vi "Actor Core.vi"(8 "error in":errorcluster, 11 "CS++BaseActor in":refnum<class "CS++BaseActor.lvclass">) -> (0 "error out":errorcluster, 3 "Actor out":refnum<class "Actor.lvclass">)   [LabVIEW 2016, in "CS++BaseActor.lvlib" / "CS++BaseActor.lvclass"]
doc: "(<B>Filename</B>: Actor Framework.lvlib:Actor.lvclass:Actor Core.vi)\n\nReceives messages to the actor, reacts to them, and initiates any error handling that may shut the actor down.\n\nDescendant classes may override this VI to append parallel tasks for the actor to complete while it handles messages. Overrides use the Call Parent Method node."
uses:
  CS++BaseActor.lvclass
  C:/Program Files (x86)/National Instruments/LabVIEW 2016/vi.lib/ActorFramework/Actor/Actor.lvclass
  <vilib>/ActorFramework/Actor/Actor.lvclass
  CS++BaseActor.lvclass/CS++BaseActor.ctl
  <vilib>/ActorFramework/Message Enqueuer/Message Priority.ctl
  <vilib>/ActorFramework/Actor/Actor.lvclass/Actor.ctl
  <vilib>/ActorFramework/Message Enqueuer/Message Enqueuer.lvclass/Message Enqueuer.ctl
  <vilib>/ActorFramework/Message Enqueuer/Enqueue.vi
  <vilib>/ActorFramework/Message Enqueuer/Init from Existing Queue.vi
  CS++BaseActor Messages/After Launch Init Msg/After Launch Init Msg.lvclass
  C:/Program Files (x86)/National Instruments/LabVIEW 2016/vi.lib/ActorFramework/Message/Message.lvclass
  <vilib>/ActorFramework/Message Priority Queue/Priority Enqueue.vi
  <vilib>/ActorFramework/Message Enqueuer/Message Enqueuer.lvclass
  Libraries/Utilities/CS++Utilities.lvlib
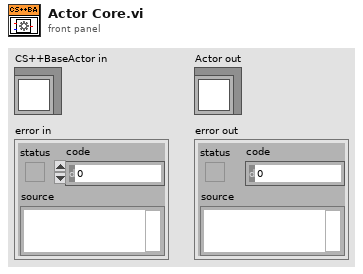
[diagram p1: front panel]
types:
  T1 = typedef "Actor Framework.lvlib/Message Enqueuer.lvclass/Message Priority.ctl" = enum16{"Low", "Normal", "High"}
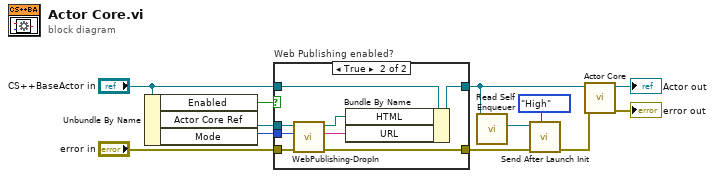
[diagram p0: block diagram]
diagram:
  n1 = Unbundle By Name("CS++BaseActor in") -> ("Enabled"=w2:bool, "Actor Core Ref"=w4:refnum<vi>, "Mode"=w3:enum16{"Snapshot", "Monitored", "Embedded"})
  n2 = case "Web Publishing enabled?" shown="True" w2 {
    tunnel: [w13 w22] -> w1
    tunnel: "error in" -> [w13 w21]
    tunnel: "CS++BaseActor in" -> [w14 w20]
    tunnel: [w14 w19] -> w5
    tunnel: w4 -> [_ w17]
    tunnel: w3 -> [_ w16]
    frame False {
    }
    frame True {
      n3 = call "WebPublishing-DropIn.vi"("Error In"=w21, "Mode (Snapshot)"=w16, "VI Ref"=w17) -> ("Error Out"=w22:errorcluster, "URL"=w18:string, "HTML File Name"=w15:path)  [unwired: 1 in, 1 out]
      n4 = Bundle By Name(cluster=w20, "HTML"=w15, "URL"=w18) -> (w19:refnum<class "CS++BaseActor.lvclass">)
    }
  }
  n5 = call <vilib>:"Read Self Enqueuer.vi"("Actor"=w5) -> ("Self Enqueuer"=w10:refnum<class "Message Enqueuer.lvclass">)  [unwired: 10 in]
  n6 = call "Send After Launch Init.vi"("Message Priority (Normal)"=Message_Priority."High", "error in (no error)"=w1, "Message Enqueuer"=w10) -> ("error out"=w8:errorcluster)  [unwired: 7 in, 1 out]
  n7 = call-parent "Actor Core.vi"("error in"=w8, "Actor in"=w5) -> ("error out"=→"error out":errorcluster, "Actor out"=→"Actor out":refnum<class "Actor.lvclass">)  [unwired: 8 in]
